vi "Update Loop Outline.vi"(10 "Start Vectors":T1, 11 "Map in":refnum<class "Maze.lvclass">) -> (3 "Map out":refnum<class "Maze.lvclass">)   [LabVIEW 2021, in "Maze.lvclass"]
uses:
  Maze.lvclass
  Position.ctl
  Maze.lvclass/Maze.ctl
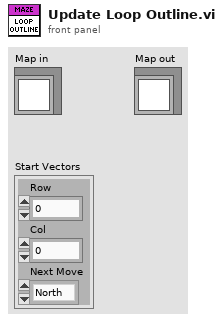
[diagram p1: front panel]
types:
  T1 = typedef "Maze.lvclass/Position.ctl" = cluster{"Row":u64, "Col":u64, "Next Move":enum16{"North", "East", "South", "West", "Halt"}}
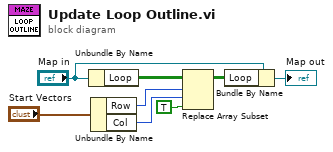
[diagram p0: block diagram]
diagram:
  n1 = Unbundle By Name("Map in") -> ("Loop"=w4:bool[][])
  n2 = Unbundle By Name("Start Vectors") -> ("Row"=w6:u64, "Col"=w7:u64)
  n3 = Replace Array Subset(array=w4, new element=TRUE ("new element/subarray"), index (row)=w6, index (col)=w7) -> (w8:bool[][])
  n4 = Bundle By Name(cluster="Map in", "Loop"=w8) -> (→"Map out":refnum<class "Maze.lvclass">)
